vi "Configure Sys (To) Clock In.vi"(7 "Level (1)":dbl=1.0 format="%#_6p", 8 "error in (no error)":errorcluster, 9 "Rate (10MHz)":dbl=10000000.0 format="%#_6p", 10 "Master Clock (F: Internal)":bool, 11 "VISA resource name":refnum<visa-resource-name>) -> (0 "error out":errorcluster, 3 "VISA resource name out":refnum<visa-resource-name>)   [LabVIEW 2012, in "Quantum Composers 9000 Series.lvlib"]
doc: "This VI is used to select the reference clock used for synchronizing the main system timer (To)."
uses:
  <instrlib>/Quantum Composers 9000 Series/Quantum Composers 9000 Series.lvlib
panel:
  # "1. The \"Rate\" and \"Level\" values are only updated\n     when an \"External\" clock source is selected.\n2. QC model 9520 only accepts clock rates of\n     10, 20, 25, 40, 50, 80, and 100MHz."
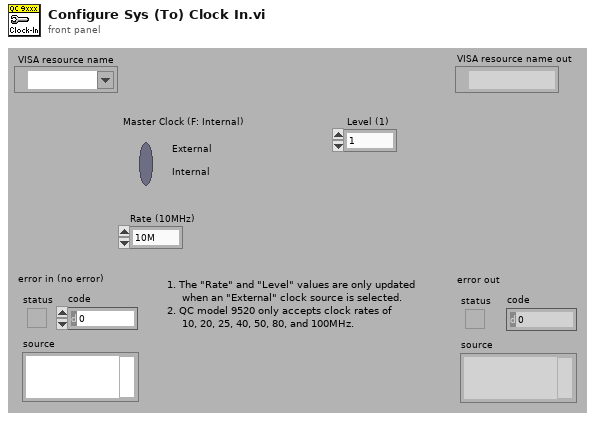
[diagram p1: front panel]
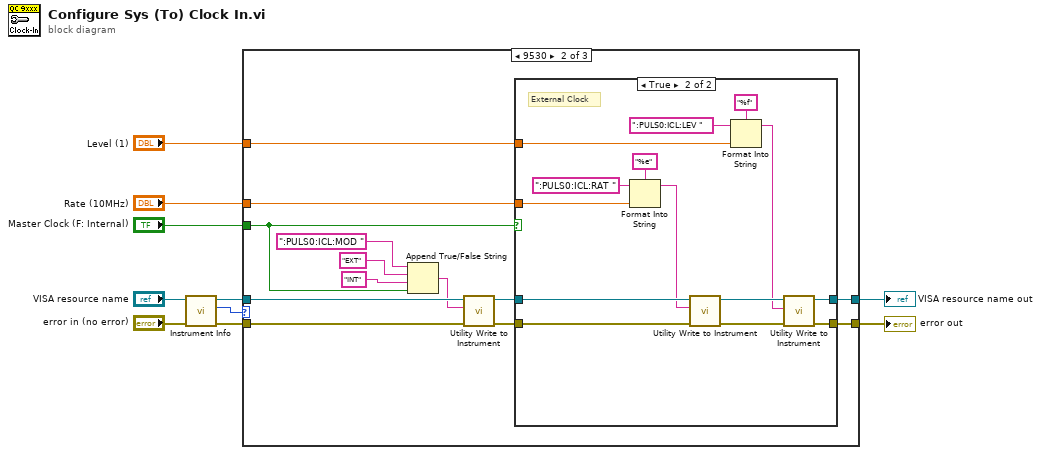
[diagram p0: block diagram]
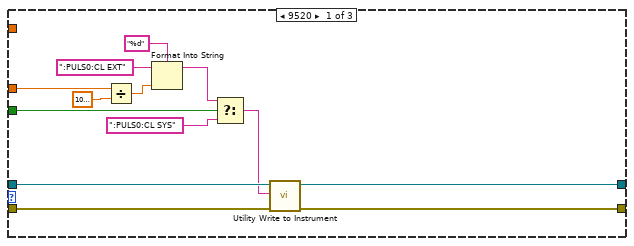
[diagram p2: hidden frame]
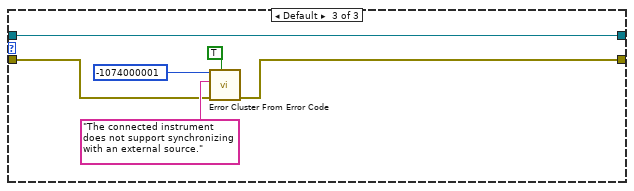
[diagram p4: hidden frame]
diagram:
  n1 = call <instrlib>:"Instrument Info.vi"("error in (no error)"="error in (no error)", "VISA resource name"="VISA resource name") -> ("error out"=w6:errorcluster, "Instr Model"=w4:u32, "VISA resource name out"=w5:refnum<visa-resource-name>)  [unwired: 6 in, 1 out]
  n2 = case shown="9530" w4 {
    tunnel: [w23 w27 w58] -> w10
    tunnel: [w22 w26 w53] -> w9
    tunnel: w6 -> [w21 w36 w54]
    tunnel: w5 -> [w20 w35 w58]
    tunnel: "Master Clock (F: Internal)" -> [w18 w28 _]
    tunnel: "Rate (10MHz)" -> [w15 w24 _]
    tunnel: "Level (1)" -> [_ w25 _]
    frame 9520 {
      n3 = Divide(x=w15, y=1000000.0) -> (x/y=w16:dbl)
      n4 = Format Into String(format string="%d", initial string=":PULS0:CL EXT", w16) -> (resulting string=w12:string)  [unwired: 1 in, 1 out]
      n5 = Select(t=w12, s=w18, f=":PULS0:CL SYS") -> (s? t:f=w11:string)
      n6 = call <instrlib>:"Utility Write to Instrument.vi"("error in (no error)"=w21, "Write Buffer"=w11, "VISA resource name"=w20) -> ("error out"=w22:errorcluster, "VISA resource name out"=w23:refnum<visa-resource-name>)  [unwired: 6 in, 1 out]
    }
    frame 9530 {
      n7 = Append True/False String(1:w28, 2:"INT" ("false string"), 3:"EXT" ("true string"), 4:":PULS0:ICL:MOD ") -> (0:w31:string)
      n8 = call <instrlib>:"Utility Write to Instrument.vi"("error in (no error)"=w36, "Write Buffer"=w31, "VISA resource name"=w35) -> ("error out"=w30:errorcluster, "VISA resource name out"=w29:refnum<visa-resource-name>)  [unwired: 6 in, 1 out]
      n9 = case shown="True" w28 {
        tunnel: w30 -> [w37 w52]
        tunnel: w29 -> [w38 w51]
        tunnel: [w38 w41] -> w27
        tunnel: [w37 w44] -> w26
        tunnel: w25 -> [_ w49]
        tunnel: w24 -> [_ w50]
        frame False {
          # "Internal Clcock"
        }
        frame True {
          # "External Clock"
          n10 = Format Into String(format string="%e", initial string=":PULS0:ICL:RAT ", w50) -> (resulting string=w39:string)  [unwired: 1 in, 1 out]
          n11 = call <instrlib>:"Utility Write to Instrument.vi"("error in (no error)"=w52, "Write Buffer"=w39, "VISA resource name"=w51) -> ("error out"=w42:errorcluster, "VISA resource name out"=w43:refnum<visa-resource-name>)  [unwired: 6 in, 1 out]
          n12 = Format Into String(format string="%f", initial string=":PULS0:ICL:LEV ", w49) -> (resulting string=w40:string)  [unwired: 1 in, 1 out]
          n13 = call <instrlib>:"Utility Write to Instrument.vi"("error in (no error)"=w42, "Write Buffer"=w40, "VISA resource name"=w43) -> ("error out"=w44:errorcluster, "VISA resource name out"=w41:refnum<visa-resource-name>)  [unwired: 6 in, 1 out]
        }
      }
    }
    frame Default {
      n14 = call <vilib>:"Error Cluster From Error Code.vi"("show call chain? (False)"=TRUE, "error in (no error)"=w54, "error message (\"\")"="The connected instrument does not support synchronizing with an external source." ("Source (VI Name)"), "error code (0)"=-1074000001 ("Code")) -> ("error out"=w53:errorcluster)  [unwired: 5 in]
    }
  }
  "error out" <- w9
  "VISA resource name out" <- w10
